vi "MetodoInit.vi"(8 "error in (no error)":errorcluster, 11 "Keysight in":refnum<class "Edu-1200.lvclass">) -> (0 "error out":errorcluster, 3 "Keysight out":refnum<class "Edu-1200.lvclass">)   [LabVIEW 2020, in "Edu-1200.lvclass"]
uses:
  Edu-1200.lvclass
  Edu-1200.lvclass/Edu-1200.ctl
  <instrlib>/Agilent 2000 3000 X-Series/Agilent 2000 3000 X-Series.lvlib
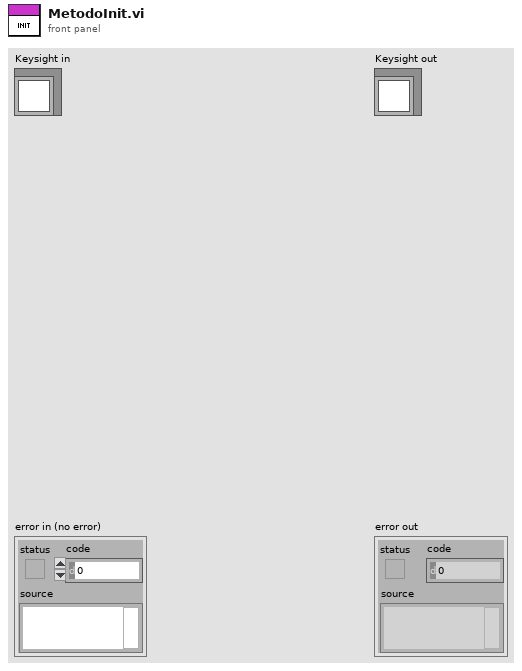
[diagram p1: front panel]
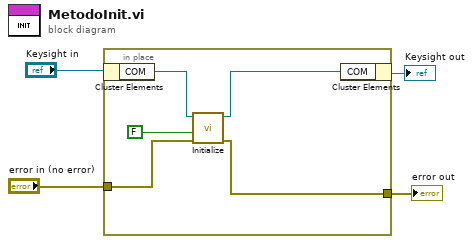
[diagram p0: block diagram]
diagram:
  n1 = in-place {
    in-place-border: "error in (no error)" -> [w9]
    in-place-border: [w8] -> w1
    n2 = in-place-cluster #1("Keysight in") -> ("COM"=w7:refnum<visa-resource-name>)
    n3 = call <instrlib>:"Initialize.vi"("error in (no error)"=w9, "Reset (True)"=FALSE, "VISA resource name"=w7) -> ("error out"=w8:errorcluster, "VISA resource name out"=w5:refnum<visa-resource-name>)  [unwired: 7 in]
    n4 = in-place-cluster #1("COM"=w5) -> (→"Keysight out":refnum<class "Edu-1200.lvclass">)
  }
  "error out" <- w1
